vi "FindTwoColorv1.vi"(4 "Friend Colors":enum32{"Pink over Green", "Green over Pink"}(radio), 6 "Color Ranges":T6(array[cluster])=[{"Hue"={"Lower"=220, "Upper"=255}, "Sat"={"Lower"=75, "Upper"=255}, " Luma"={"Lower"=85, "Upper"=255}}, {"Hue"={"Lower"=55, "Upper"=125}, "Sat"={"Lower"=58, "Upper"=255}, " Luma"={"Lower"=92, "Upper"=255}}], 7 "Adv Processing Data":T3={"SubRect"={"Left"=0, "Top"=0, "Right"=640, "Bottom"=480}, "Decimate"={"H"=2, "V"=2}}, 8 "Processing Data":T5={" Limits"={"Find Foe"=TRUE, "Max Time (sec)"=0.25, "Min Particle Size %"=0.005, "Max Particles"=10}, "Image Size"=enum."320x240", "Pink First"=TRUE}, 9 "Color Image In":T2) -> (0 "Track Time":u32, 1 "Found":bool, 2 "Target":T1, 3 "Mask Image":T2)   [LabVIEW 2013]
doc: "This VI locates areas of the image which contain both colors, one directly above the other. It can return the location of the largest friend or foe. Be sure to pay attention to the found output as well."
uses:
  <vilib>/vision/Image Controls.llb/IMAQ Image.ctl
  <vilib>/Rock Robotics/WPI/Camera/WPI_CameraImageSize.ctl
  Team Designationv1.ctl
  <vilib>/vision/NI_Vision_Development_Module.lvlib
panel:
  out "HSL Image for debugging and calibration":T2(plugin-control)
  in  "HSL Debug":bool
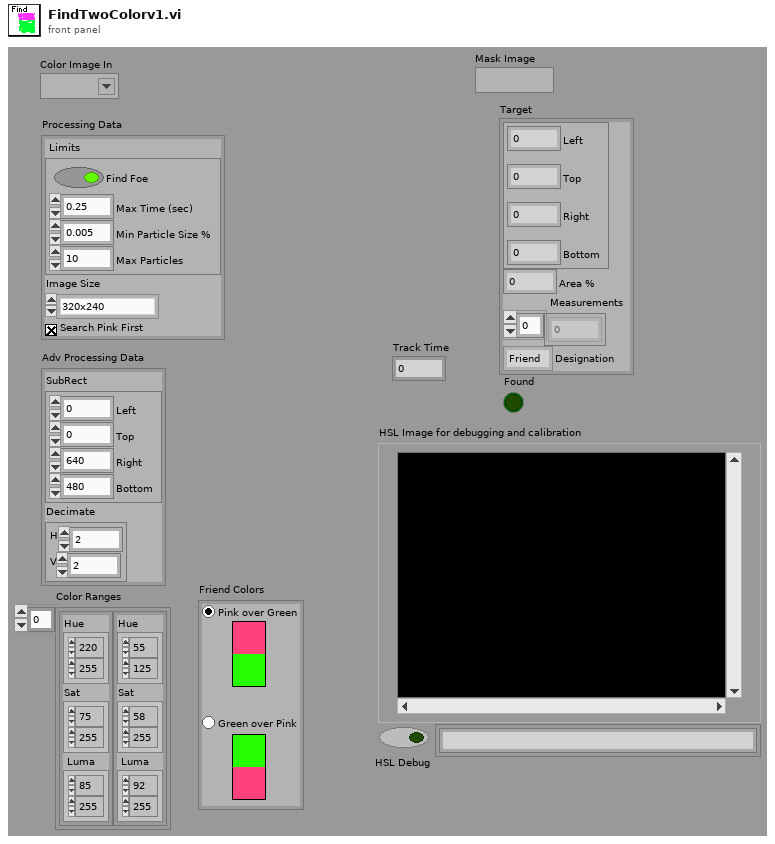
[diagram p1: front panel]
types:
  T1 = cluster{"Rectangle":cluster{"Left":i32, "Top":i32, "Right":i32, "Bottom":i32}, "Area %":dbl, "Measurements":dbl[], "Designation":enum16{"Friend", "Foe"}}
  T2 = typedef "IMAQ Image.ctl" = refnum<image>
  T3 = cluster{"SubRect":cluster{"Left":i32, "Top":i32, "Right":i32, "Bottom":i32}, "Decimate":cluster{"H":i32, "V":i32}}
  T4 = typedef "WPI_CameraImageSize.ctl" = enum16{"640x480", "320x240", "160x120"}
  T5 = cluster{" Limits":cluster{"Find Foe":bool, "Max Time (sec)":dbl, "Min Particle Size %":sgl, "Max Particles":i32}, "Image Size":T4, "Pink First":bool}
  T6 = cluster{"Hue":cluster{"Lower":i32, "Upper":i32}, "Sat":cluster{"Lower":i32, "Upper":i32}, " Luma":cluster{"Lower":i32, "Upper":i32}}[]
  T7 = cluster{"HSL Image":T2, "Subset Image":T2, "AboveSub Image":T2, "BelowSub Image":T2, "AboveSub ImageHSL":T2, "BelowSub ImageHSL":T2, "Mask Above Image":T2, "BelowMask Image":T2, "Mask Image":T2}
  T8 = cluster{"Left":i32, "Top":i32, "Right":i32, "Bottom":i32}
  T9 = cluster{"Left":i32, "Top":i32, "Left":i32, "Top":i32}
  T10 = typedef "Image Type" = u32
  T11 = cluster{"Find Foe":bool, "Max Time (sec)":dbl, "Min Particle Size %":sgl, "Max Particles":i32}
  T12 = cluster{"Pink First":bool, "Friend Colors":enum32{"Pink over Green", "Green over Pink"}}
  T13 = cluster{"Hue":cluster{"Lower":i32, "Upper":i32}, "Sat":cluster{"Lower":i32, "Upper":i32}, " Luma":cluster{"Lower":i32, "Upper":i32}}
  T14 = cluster{"Pixel Area":dbl, "Rectangle":cluster{"Left":i32, "Top":i32, "Right":i32, "Bottom":i32}, "Additional Measurements":dbl[]}[]
  T15 = typedef "Team Designationv1.ctl" = enum16{"FoS", "SoF"}
  T16 = cluster{"left":i32, "top":i32, "right":i32, "bottom":i32}
  T17 = cluster{cluster{i32, i32, i32, i32}, dbl, "Target Designation":T15, "Additional Measurements":dbl[]}
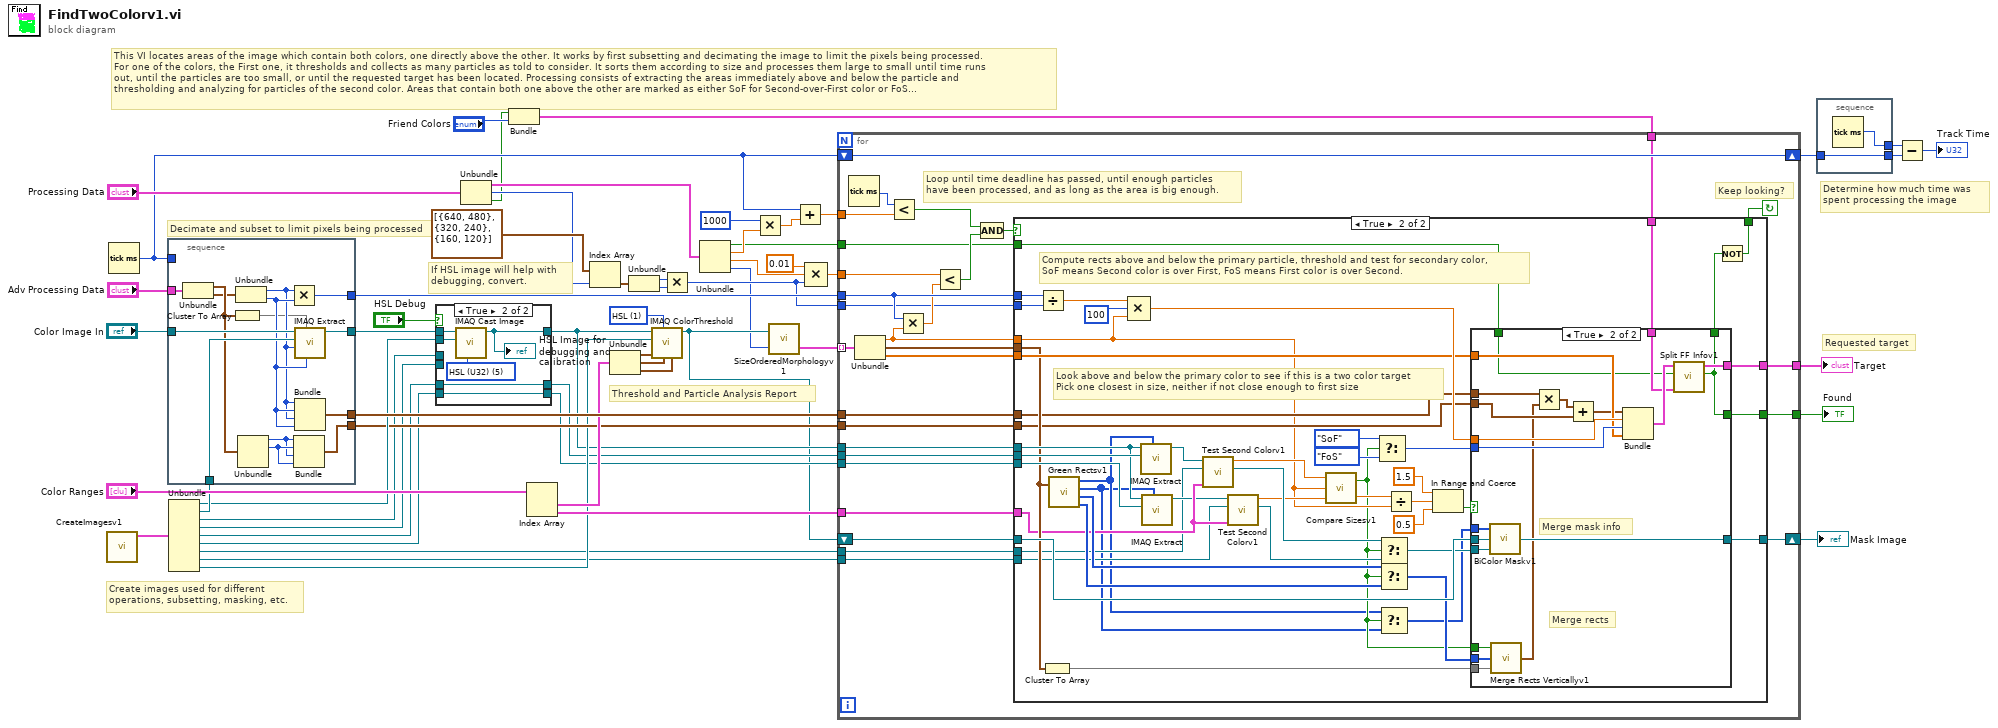
[diagram p0: block diagram]
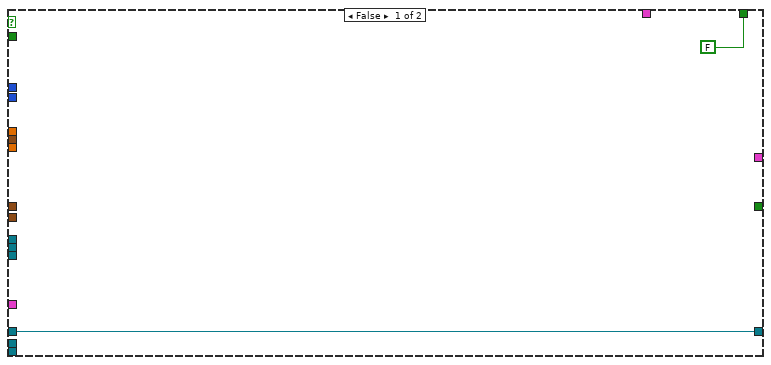
[diagram p3: hidden frame]
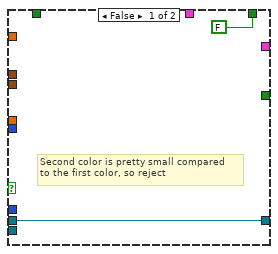
[diagram p4: hidden frame]
diagram:
  w53 = u16 1 items=["RGB", "HSL", "HSV", "HSI"] ("Color Mode")
  # "Requested target"
  # "Determine how much time was\nspent processing the image"
  # "Create images used for different\noperations, subsetting, masking, etc."
  # "Threshold and Particle Analysis Report"
  # "If HSL image will help with\ndebugging, convert."
  # "Decimate and subset to limit pixels being processed"
  # "This VI locates areas of the image which contain both colors, one directly above the other. It works by first subsetting and decimating the image to limit the pixels being processed.\nFor one of the colors, the First one, it thresholds and collects as many particles as told to consider. It sorts them according to size and processes them large to small until time runs\nout, until the particles are too small, or until the requested target has been located. Processing consists of extracting the areas immediately above and below the particle and\nthresholding and analyzing for particles of the second color. Areas that contain both one above the other are marked as either SoF for Second-over-First color or FoS..."
  n1 = call "CreateImagesv1.vi"() -> ("Images"=w43:T7)  [unwired: 11 out]
  n2 = Tick Count (ms)() -> (millisecond timer value=w13:u32)
  n3 = Unbundle(w43) -> ("HSL Image"=w41:T2, "Subset Image"=w42:T2, "AboveSub Image"=w23:T2, "BelowSub Image"=w21:T2, "AboveSub ImageHSL"=w25:T2, "BelowSub ImageHSL"=w24:T2, "Mask Above Image"=w26:T2, "BelowMask Image"=w27:T2, "Mask Image"=w28:T2)
  n4 = stacked-sequence {
    tunnel: "Color Image In" -> [w71]
    tunnel: [w69] -> w44
    tunnel: w42 -> [w70]
    tunnel: [w68] -> w51
    tunnel: [w66] -> w52
    tunnel: [w61] -> w30
    tunnel: "Adv Processing Data" -> [w60]
    tunnel: w13 -> [_]
    frame #0 {
      n5 = Unbundle(w60) -> ("SubRect"=w59:T8, "Decimate"=w58:cluster{"H":i32, "V":i32})
      n6 = Cluster To Array(cluster=w59) -> (array=w64:i32[])
      n7 = Unbundle(w58) -> ("H"=w65:i32, "V"=w67:i32)
      n8 = Unbundle(w59) -> ("Left"=w62:i32, "Top"=w63:i32)  [unwired: 2 out]
      n9 = Multiply(x=w65, y=w67) -> (x*y=w68:i32)
      n10 = Bundle("Left"=w62, "Top"=w63, "Left"=w62, "Top"=w63) -> (w61:T9)  [unwired: 1 out]
      n11 = call "IMAQ Extract"("Y Step Size"=w67, "Optional Rectangle"=w64, "X Step Size"=w65, "Image Dst"=w70, "Image Src"=w71) -> ("Image Dst Out"=w69:T2)  [unwired: 1 in, 5 out]
      n12 = Bundle("H"=w65, "V"=w67, "H"=w65, "V"=w67) -> (w66:cluster{"H":i32, "V":i32, "H":i32, "V":i32})  [unwired: 1 out]
    }
  }
  n13 = case shown="True" "HSL Debug" {
    tunnel: [w74 w75] -> w14
    tunnel: w44 -> [w74 w80]
    tunnel: w41 -> [_ w79]
    tunnel: w23 -> [w73 _]
    tunnel: w21 -> [w72 _]
    tunnel: w25 -> [_ w77]
    tunnel: w24 -> [_ w78]
    tunnel: [w73 w77] -> w22
    tunnel: [w72 w78] -> w20
    frame False {
    }
    frame True {
      w76 = T10 5 items=["Grayscale (U8)", "Grayscale (I16)", "Grayscale (SGL)", "Complex (CSG)", "RGB (U32)", "HSL (U32)", "RGB (U64)"] ("Image Type")
      n14 = call "IMAQ Cast Image"("Image Type"=w76, "Image Dst"=w79, "Image Src"=w80) -> ("Image Dst Out"=w75:T2)  [unwired: 3 in, 5 out]
      "HSL Image for debugging and calibration" <- w75
    }
  }
  n15 = Unbundle("Processing Data") -> ("Limits"=w37:T11, "Image Size"=w34:T4, "Pink First"=w8:bool)
  n16 = Bundle("Pink First"=w8, "Friend Colors"="Friend Colors") -> (w7:T12)  [unwired: 1 out]
  n17 = Index Array(array="Color Ranges") -> (element #1=w47:T13, element #2=w46:T13)  [unwired: 2 in]
  n18 = Index Array(array=cluster{"X":i32, "Y":i32}[] [{"X"=640, "Y"=480}, {"X"=320, "Y"=240}, {"X"=160, "Y"=120}] ("Resolutions"), index=w34) -> (element=w33:cluster{"X":i32, "Y":i32})
  n19 = Unbundle(w47) -> ("Hue"=w48:cluster{"Lower":i32, "Upper":i32}, "Sat"=w50:cluster{"Lower":i32, "Upper":i32}, "Luma"=w49:cluster{"Lower":i32, "Upper":i32})
  n20 = Unbundle(w33) -> ("X"=w19:i32, "Y"=w18:i32)
  n21 = call "IMAQ ColorThreshold"("Blue or Luma or Val or Inten Range"=w49, "Green or Sat Range"=w50, "Color Mode"=w53, "Red or Hue Range"=w48, "Image Dst"=w28, "Image Src"=w14) -> ("Image Dst Out"=w12:T2)  [unwired: 2 in, 3 out]
  n22 = Multiply(x=w19, y=w18) -> (x*y=w17:i32)
  n23 = Unbundle(w37) -> ("Find Foe"=w2:bool, "Max Time (sec)"=w4:dbl, "Min Particle Size %"=w3:sgl, "Max Particles"=w5:i32)
  n24 = Multiply(x=1000, y=w4) -> (x*y=w15:dbl)
  n25 = call "SizeOrderedMorphologyv1.vi"("Report Size Limit"=w5, "Image Dst Out"=w12) -> ("Particles"=w45:T14)  [unwired: 1 out]
  n26 = Add(x=w13, y=w15) -> (x+y=w39:dbl)
  n27 = Compound Arithmetic op=MULTIPLY(0.01, w3, w17) -> (w36:dbl)
  n28 = for {
    tunnel: w52 -> [w103]
    tunnel: w51 -> [w96]
    tunnel: w45 -> [w109] mode=indexing
    tunnel: w46 -> [w105]
    tunnel: w14 -> [w107]
    tunnel: w22 -> [w108]
    tunnel: w20 -> [w106]
    tunnel: w26 -> [w82]
    tunnel: w27 -> [w81]
    tunnel: w39 -> [w98]
    tunnel: w36 -> [w101]
    tunnel: w30 -> [w94]
    shift-right: [w102] -> w40
    shift-left: w13 -> [w102]
    tunnel: w17 -> [w93]
    shift-right: [w90] -> w11
    shift-left: w12 -> [w91]
    tunnel: w7 -> [w88]
    tunnel: [w86] -> w6
    tunnel: w2 -> [w84]
    tunnel: [w83] -> w1
    stop <- w85 continue-if-true
    # "Keep looking?"
    # "Loop until time deadline has passed, until enough particles\nhave been processed, and as long as the area is big enough."
    n29 = Tick Count (ms)() -> (millisecond timer value=w99:u32)
    n30 = Unbundle(w109) -> ("Pixel Area"=w97:dbl, "Rectangle"=w104:T8, "Additional Measurements"=w92:dbl[])
    n31 = Less?(x=w99, y=w98) -> (x < y?=w89:bool)
    n32 = Multiply(x=w96, y=w97) -> (x*y=w95:dbl)
    n33 = Less?(x=w101, y=w95) -> (x < y?=w87:bool)
    n34 = Compound Arithmetic op=AND(w89, w87) -> (w100:bool)
    n35 = case shown="True" w100 {
      tunnel: w96 -> [_ w150]
      tunnel: w108 -> [_ w158]
      tunnel: w107 -> [_ w157]
      tunnel: w106 -> [_ w156]
      tunnel: w105 -> [_ w121]
      tunnel: w97 -> [_ w118]
      tunnel: w104 -> [_ w142]
      tunnel: w103 -> [_ w140]
      tunnel: w94 -> [_ w141]
      tunnel: w93 -> [_ w149]
      tunnel: w92 -> [_ w147]
      tunnel: w91 -> [w111 w146]
      tunnel: [w111 w145] -> w90
      tunnel: w88 -> [_ w136]
      tunnel: [_ w135] -> w86
      tunnel: [FALSE w132] -> w85
      tunnel: w84 -> [_ w134]
      tunnel: [_ w131] -> w83
      tunnel: w82 -> [_ w117]
      tunnel: w81 -> [_ w116]
      frame False {
      }
      frame True {
        # "Compute rects above and below the primary particle, threshold and test for secondary color,\nSoF means Second color is over First, FoS means First color is over Second."
        # "Look above and below the primary color to see if this is a two color target\nPick one closest in size, neither if not close enough to first size"
        n36 = Divide(x=w150, y=w149) -> (x/y=w148:dbl)
        n37 = Cluster To Array(cluster=w142) -> (array=w138:i32[])
        n38 = call "Green Rectsv1.vi"("Rectangle"=w142) -> ("Test Upper"=w114:i32[], "Test Lower"=w113:i32[], "Orig Upper"=w125:i32[], "Orig Lower"=w124:i32[])  [unwired: 1 in]
        n39 = Compound Arithmetic op=MULTIPLY(w148, 100, w118) -> (w154:dbl)
        n40 = call "IMAQ Extract"("Optional Rectangle"=w114, "Image Dst"=w158, "Image Src"=w157) -> ("Image Dst Out"=w119:T2)  [unwired: 3 in, 5 out]
        n41 = call "IMAQ Extract"("Optional Rectangle"=w113, "Image Dst"=w156, "Image Src"=w157) -> ("Image Dst Out"=w120:T2)  [unwired: 3 in, 5 out]
        n42 = call "Test Second Colorv1.vi"("Image"=w119, "Mask Image"=w117, "Color Ranges"=w121) -> ("Pixel Area"=w126:dbl, "Image Dst Out"=w144:T2)  [unwired: 1 in, 4 out]
        n43 = call "Test Second Colorv1.vi"("Image"=w120, "Mask Image"=w116, "Color Ranges"=w121) -> ("Pixel Area"=w123:dbl, "Image Dst Out"=w122:T2)  [unwired: 5 out]
        n44 = call "Compare Sizesv1.vi"("Below Area"=w123, "First  Area"=w118, "Above Area"=w126) -> ("Closest Area"=w155:dbl, "Above?"=w115:bool)
        n45 = Select(t=Team_Designationv1."SoF" ("Target Designation"), s=w115, f=Team_Designationv1."FoS" ("Target Designation")) -> (s? t:f=w151:T15)
        n46 = Select(t=w144, s=w115, f=w122) -> (s? t:f=w143:T2)
        n47 = Select(t=w125, s=w115, f=w124) -> (s? t:f=w139:i32[])
        n48 = Select(t=w114, s=w115, f=w113) -> (s? t:f=w112:i32[])
        n49 = Divide(x=w155, y=w118) -> (x/y=w129:dbl)
        n50 = In Range and Coerce(upper limit=1.5, x=w129, lower limit=0.5) -> (In Range?=w130:bool)  [unwired: 1 out]
        n51 = case shown="True" w130 {
          tunnel: w154 -> [_ w180]
          tunnel: w151 -> [_ w179]
          tunnel: w147 -> [_ w178]
          tunnel: w146 -> [w160 w177]
          tunnel: w112 -> [_ w176]
          tunnel: [w160 w175] -> w145
          tunnel: w143 -> [_ w174]
          tunnel: w141 -> [_ w172]
          tunnel: w140 -> [_ w171]
          tunnel: w115 -> [_ w168]
          tunnel: w139 -> [_ w167]
          tunnel: w138 -> [_ w166]
          tunnel: w136 -> [_ w164]
          tunnel: [_ w162] -> w135
          tunnel: w134 -> [_ w163]
          tunnel: [FALSE w161] -> w133
          tunnel: [_ w161] -> w131
          frame False {
            # "Second color is pretty small compared\nto the first color, so reject"
          }
          frame True {
            # "Merge rects"
            # "Merge mask info"
            n52 = call "BiColor Maskv1.vi"("Second Mask"=w174, "First Mask"=w177, "Rectangle"=w176) -> ("Image Dst Out"=w175:T2)
            n53 = call "Merge Rects Verticallyv1.vi"("First"=w166, "Second"=w167, "Above"=w168) -> ("Rect"=w169:T16)
            n54 = Multiply(x=w171, y=w169) -> (x*y=w173:cluster{i32, i32, i32, i32})
            n55 = Add(x=w173, y=w172) -> (x+y=w170:cluster{i32, i32, i32, i32})
            n56 = Bundle(w170, w180, "Target Designation"=w179, "Additional Measurements"=w178) -> (w165:T17)  [unwired: 1 out]
            n57 = call "Split FF Infov1.vi"("Team Color Info"=w164, "Find Foe"=w163, "Target"=w165) -> ("Found"=w161:bool, "Target out"=w162:T1)  [unwired: 3 out]
          }
        }
        n58 = Not(x=w133) -> (.not. x?=w132:bool)
      }
    }
  }
  "Mask Image" <- w11
  "Target" <- w6
  "Found" <- w1
  n59 = stacked-sequence {
    tunnel: [w182] -> w57
    tunnel: w40 -> [w182]
    tunnel: [w181] -> w56
    frame #0 {
      n60 = Tick Count (ms)() -> (millisecond timer value=w181:u32)
    }
  }
  n61 = Subtract(x=w56, y=w57) -> (x-y=→"Track Time":u32)
